vi "Query RX labels for Params.vi"(8 "error in":errorcluster, 11 "node result array":refnum<k20>[](array[refnum])) -> (0 "error out":errorcluster, 3 "LabelParams":T1[](array[typedef]))   [LabVIEW 2016]
uses:
  Controls/LabelParam.ctl
  Controls/LabelInfo.ctl
  Controls/ARINCParam.ctl
  <vilib>/xml/Close Reference(Node).vi
  <vilib>/xml/Close Reference(NNMap).vi
  Ballard Arinc-429 System Explorer.lvlib
  <resource>/objmgr/DOMUserDefRef.rc
  <vilib>/xml/NI_XML.lvlib
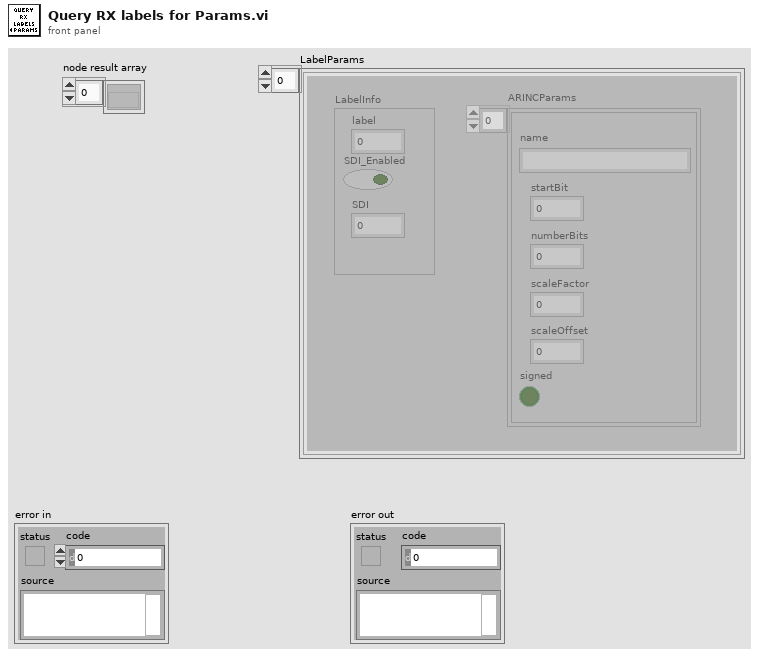
[diagram p1: front panel]
types:
  T1 = typedef "Ballard Arinc-429 System Explorer.lvlib/LabelParam.ctl" = cluster{"LabelInfo":T2, "ARINCParams":T3[]}
  T2 = typedef "Ballard Arinc-429 System Explorer.lvlib/LabelInfo.ctl" = cluster{"label":u32, "SDI_Enabled":bool, "SDI":u8}
  T3 = typedef "Ballard Arinc-429 System Explorer.lvlib/ARINCParam.ctl" = cluster{"name":string, "startBit":i32, "numberBits":i32, "scaleFactor":dbl, "scaleOffset":dbl, "signed":bool}
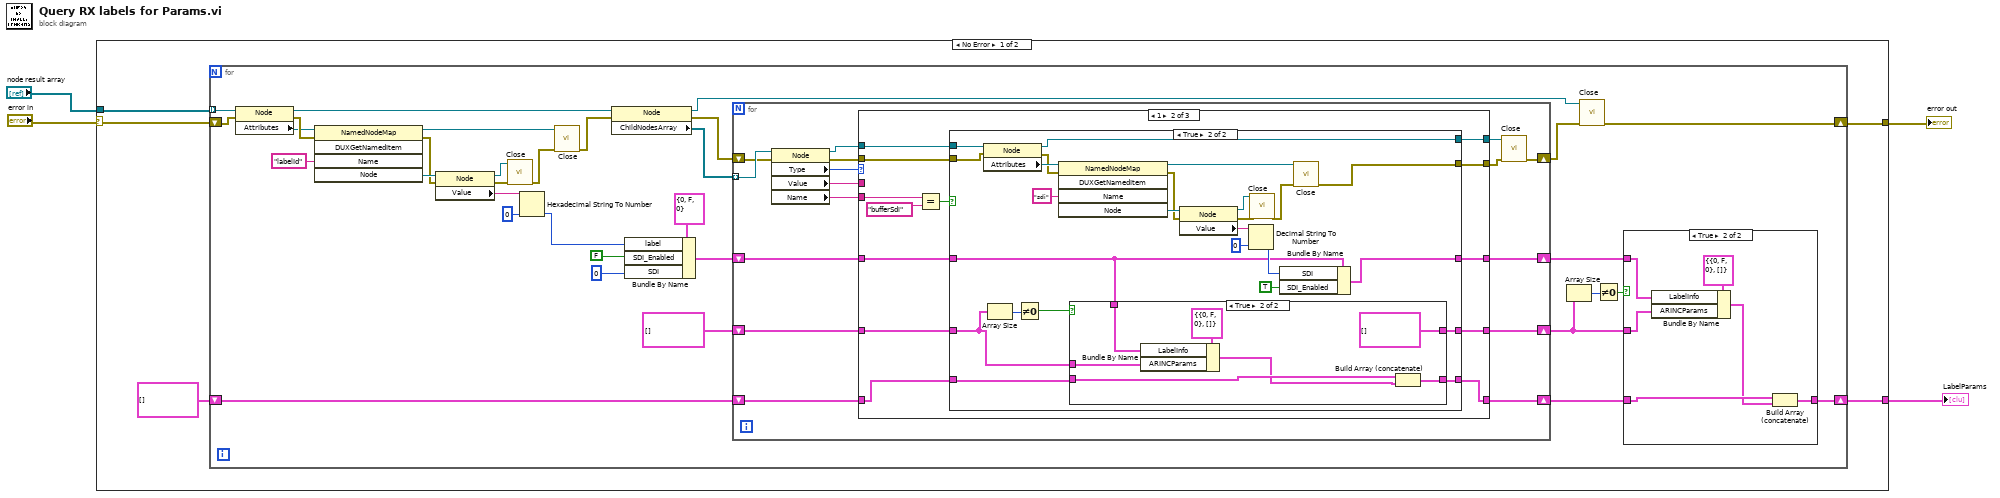
[diagram p0: block diagram]
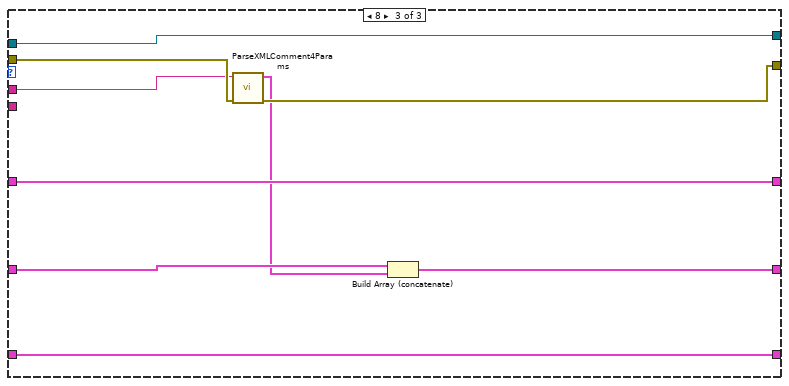
[diagram p6: hidden frame]
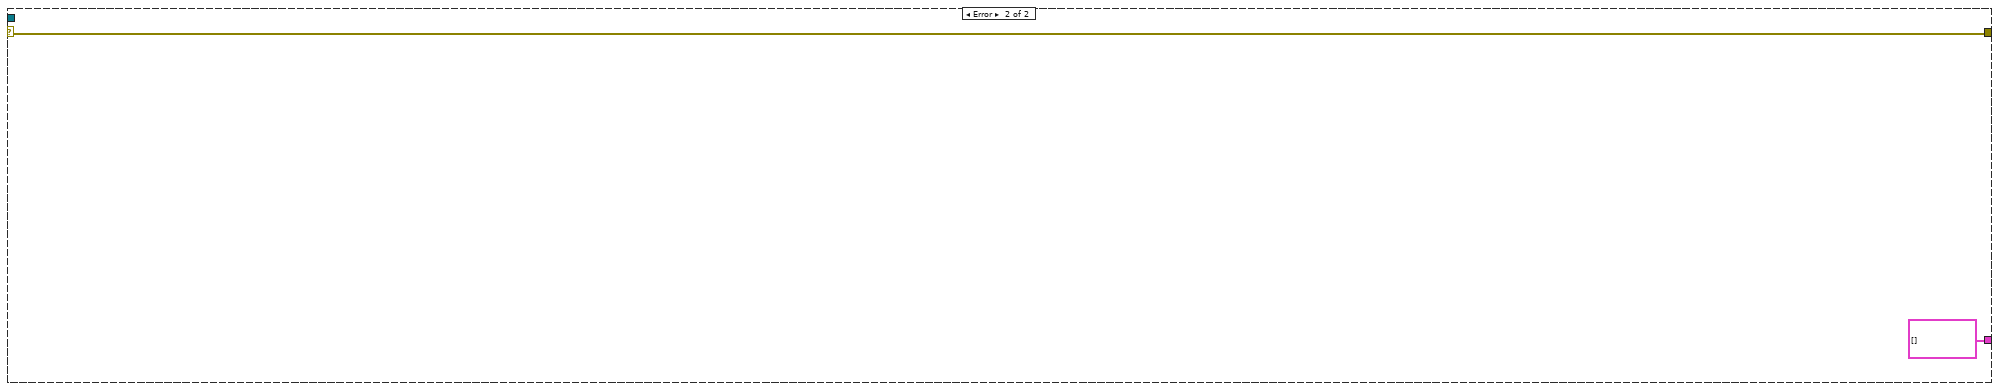
[diagram p7: hidden frame]
diagram:
  n1 = case shown="No Error" "error in" {
    selector: "error in" -> [w5 w133]
    tunnel: "node result array" -> [w8 _]
    tunnel: [w7 T1[] []] -> w3
    tunnel: [w6 w133] -> w2
    frame No Error {
      n2 = for {
        tunnel: w8 -> [w18] mode=indexing
        shift-right: [w40] -> w6
        shift-left: w5 -> [w17]
        shift-right: [w11] -> w7
        shift-left: T1[] [] -> [w19]
        n3 = property class="Node"(reference=w18, error in=w17) -> (reference out=w37:refnum<k20>, error out=w36:errorcluster, "Attributes"=w35:refnum<k20>)
        n4 = invoke class="NamedNodeMap" method="DUXGetNamedItem"(reference=w35, error in=w36, "Name"="labelId") -> (reference out=w29:refnum<k20>, error out=w32:errorcluster, "Node"=w33:refnum<k20>)  [unwired: 2 in, 2 out]
        n5 = property class="Node"(reference=w33, error in=w32) -> (reference out=w31:refnum<k20>, error out=w30:errorcluster, "Value"=w26:string)
        n6 = call-poly <vilib>:"Close.vi"("error in (no error)"=w30, "node"=w31) -> ("error out"=w28:errorcluster)  [unwired: 7 out]
        n7 = Hexadecimal String To Number(string=w26, default (0uL)=u32 0 ("default (0 I32)")) -> (number=w25:u32)  [unwired: 1 in, 1 out]
        n8 = call-poly <vilib>:"Close.vi"("error in (no error)"=w28, "named node map"=w29) -> ("error out"=w27:errorcluster)  [unwired: 7 out]
        n9 = property class="Node"(reference=w37, error in=w27) -> (reference out=w39:refnum<k20>, error out=w41:errorcluster, "ChildNodesArray"=w42:refnum<k20>[])
        n10 = Bundle By Name(cluster=T2 {"label"=0, "SDI_Enabled"=FALSE, "SDI"=0} ("output cluster"), "label"=w25, "SDI_Enabled"=FALSE, "SDI"=u8 0 ("default (0 I32)")) -> (w21:T2)
        n11 = for {
          tunnel: w42 -> [w65] mode=indexing
          shift-right: [w60] -> w38
          shift-left: w41 -> [w64]
          shift-right: [w55] -> w10
          shift-left: w21 -> [w56]
          shift-right: [w53] -> w12
          shift-left: w19 -> [w54]
          shift-right: [w51] -> w13
          shift-left: T3[] [] -> [w52]
          n12 = property class="Node"(reference=w65, error in=w64) -> (reference out=w58:refnum<k20>, error out=w61:errorcluster, "Type"=w63:i32, "Value"=w62:string, "Name"=w50:string)
          n13 = case shown="1" w63 {
            tunnel: w62 -> [_ _ w130]
            tunnel: w61 -> [w70 w81 w131]
            tunnel: [w70 w80 w129] -> w59
            tunnel: w58 -> [w67 w83 w128]
            tunnel: [w67 w82 w128] -> w57
            tunnel: w56 -> [w69 w76 w127]
            tunnel: [w69 w79 w127] -> w55
            tunnel: w54 -> [w68 w78 w123]
            tunnel: [w68 w77 w123] -> w53
            tunnel: w52 -> [w66 w75 w126]
            tunnel: [w66 w74 w124] -> w51
            tunnel: w50 -> [_ w73 _]
            frame 0, Default {
            }
            frame 1 {
              n14 = Equal?(x=w73, y="bufferSdi" ("sdiITagName")) -> (x = y?=w71:bool)
              n15 = case shown="True" w71 {
                tunnel: w83 -> [w84 w113]
                tunnel: [w84 w112] -> w82
                tunnel: w81 -> [w85 w111]
                tunnel: [w85 w101] -> w80
                tunnel: [w88 w96] -> w79
                tunnel: w78 -> [w86 w93]
                tunnel: [w86 w92] -> w77
                tunnel: w76 -> [w88 w91]
                tunnel: w75 -> [w87 w90]
                tunnel: [w87 w89] -> w74
                frame False {
                }
                frame True {
                  n16 = property class="Node"(reference=w113, error in=w111) -> (reference out=w112:refnum<k20>, error out=w108:errorcluster, "Attributes"=w110:refnum<k20>)
                  n17 = Array Size(array=w90) -> (size(s)=w95:i32)
                  n18 = Not Equal To 0?(x=w95) -> (x != 0?=w94:bool)
                  n19 = invoke class="NamedNodeMap" method="DUXGetNamedItem"(reference=w110, error in=w108, "Name"="sdi") -> (reference out=w103:refnum<k20>, error out=w106:errorcluster, "Node"=w107:refnum<k20>)  [unwired: 2 in, 2 out]
                  n20 = case shown="True" w94 {
                    tunnel: w93 -> [w115 w122]
                    tunnel: [w115 w121] -> w92
                    tunnel: w91 -> [_ w118]
                    tunnel: w90 -> [w114 w117]
                    tunnel: [w114 T3[] []] -> w89
                    frame False {
                    }
                    frame True {
                      n21 = Bundle By Name(cluster=T1 {"LabelInfo"={"label"=0, "SDI_Enabled"=FALSE, "SDI"=0}, "ARINCParams"=[]} ("LabelParam"), "LabelInfo"=w118, "ARINCParams"=w117) -> (w119:T1)
                      n22 = Build Array (concatenate)(w122, w119) -> (w121:T1[])
                    }
                  }
                  n23 = property class="Node"(reference=w107, error in=w106) -> (reference out=w104:refnum<k20>, error out=w105:errorcluster, "Value"=w97:string)
                  n24 = Decimal String To Number(string=w97, default (0L)=u8 0 ("default (0 I32)")) -> (number=w100:u8)  [unwired: 1 in, 1 out]
                  n25 = call-poly <vilib>:"Close.vi"("error in (no error)"=w105, "node"=w104) -> ("error out"=w102:errorcluster)  [unwired: 7 out]
                  n26 = Bundle By Name(cluster=w91, "SDI"=w100, "SDI_Enabled"=TRUE) -> (w96:T2)
                  n27 = call-poly <vilib>:"Close.vi"("error in (no error)"=w102, "named node map"=w103) -> ("error out"=w101:errorcluster)  [unwired: 7 out]
                }
              }
            }
            frame 8 {
              n28 = call "ParseXMLComment4Params.vi"("error in"=w131, "XML Comment"=w130) -> ("error out"=w129:errorcluster, "ARINC Parameter"=w125:T3)  [unwired: 8 in]
              n29 = Build Array (concatenate)(w126, w125) -> (w124:T3[])
            }
          }
          n30 = call-poly <vilib>:"Close.vi"("error in (no error)"=w59, "node"=w57) -> ("error out"=w60:errorcluster)  [unwired: 7 out]
        }
        n31 = Array Size(array=w13) -> (size(s)=w15:i32)
        n32 = call-poly <vilib>:"Close.vi"("error in (no error)"=w38, "node"=w39) -> ("error out"=w40:errorcluster)  [unwired: 7 out]
        n33 = Not Equal To 0?(x=w15) -> (x != 0?=w14:bool)
        n34 = case shown="True" w14 {
          tunnel: w13 -> [_ w47]
          tunnel: w12 -> [w43 w45]
          tunnel: [w43 w46] -> w11
          tunnel: w10 -> [_ w48]
          frame False {
          }
          frame True {
            n35 = Bundle By Name(cluster=T1 {"LabelInfo"={"label"=0, "SDI_Enabled"=FALSE, "SDI"=0}, "ARINCParams"=[]} ("LabelParam"), "LabelInfo"=w48, "ARINCParams"=w47) -> (w44:T1)
            n36 = Build Array (concatenate)(w45, w44) -> (w46:T1[])
          }
        }
      }
    }
    frame Error {
    }
  }
  "LabelParams" <- w3
  "error out" <- w2
